vi "createResultsRowLinear.vi"(6 "Indices to Output":bool[](array[boolean]), 7 "Analysis Info cluster":T2[](array[typedef]) {"Sync Delay Time (s)" format="%.4f"; "Total Meas Time (s)" format="%_5g"; "Sd Error in Variance" format="%_3g"; "Skew_u" format="%_3g"; "% u'/U" format="%_3g"; "Sd Error in Mean" format="%_3g"; "Kurt_u" format="%_3g"; "u^4" format="%_3g"; "u^3" format="%_3g"; "U" format="%_3g"; "u^2" format="%_3g"}, 8 "Error String":string, 9 "MetadataValuesIn":string[](array[string]), 11 "MetadataNamesIn":string[](array[string])) -> (0 "row splitting":string[][](array[string]), 1 "Ch Values Out":string[](array[string]), 3 "Ch Names Out":string[](array[string]), 4 "Values to Keep in Dup rows":bool[](array[boolean]))   [LabVIEW 2022 SP3]
uses:
  Controls/Analysis_info_cluster.ctl
  Controls/Inst_type.ctl
  Controls/Instrument_Array.ctl
  Controls/channelState.ctl
  Globals/Dynamic_call_global.ph.vi
panel:
  out "ScrollableArray":T1(array[cluster])
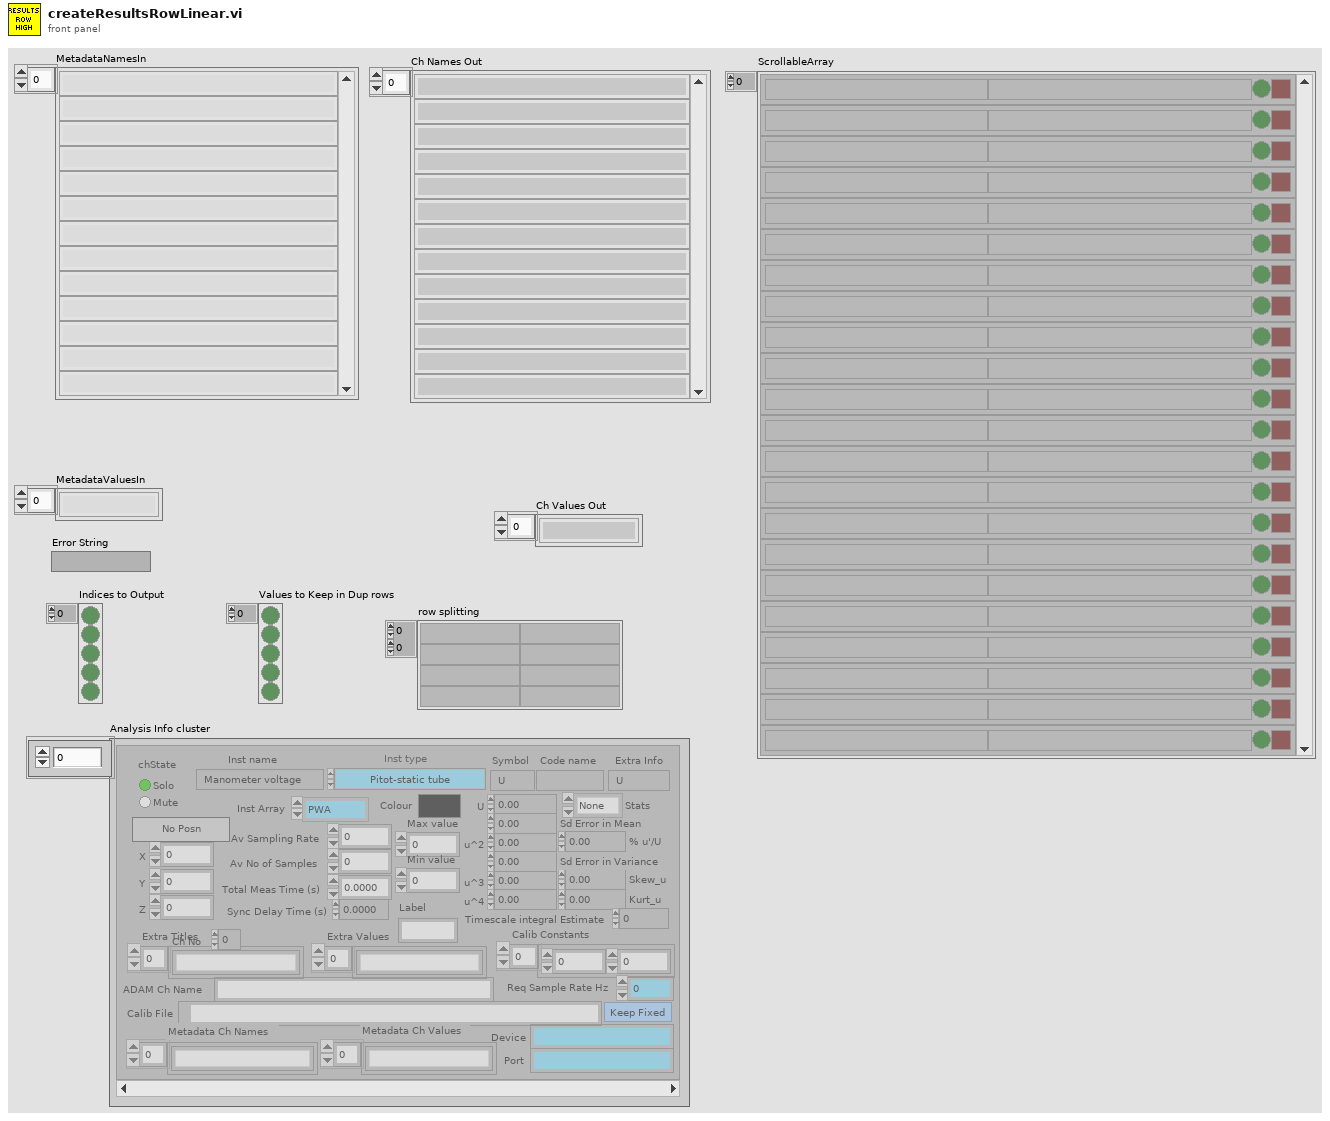
[diagram p1: front panel]
types:
  T1 = cluster{"Input Element":string, "name":string, bool, bool}[]
  T2 = typedef "Analysis_info_cluster.ctl" = cluster{"Colour":u32, "Inst type":T3, "Inst name":string, "Symbol":string, "Code name":string, "Extra Info":string, "Inst Array":T4, "Extra Titles":string[], "Extra Values":string[], "U":dbl, "u^2":dbl, "u^3":dbl, "u^4":dbl, "Skew_u":dbl, "Kurt_u":dbl, "Sd Error in Mean":dbl, "% u'/U":dbl, "X":dbl, "Y":dbl, "Z":dbl, "Timescale integral Estimate":dbl, "Sd Error in Variance":dbl, "Calib File":path, "Calib Constants":dbl[], "Output Position":bool, "Stats":enum16{"None", "Basic", "Full"}, "Av Sampling Rate":dbl, "Av No of Samples":dbl, "Total Meas Time (s)":dbl, "ADAM Ch Name":string, "Max value":dbl, "Min value":dbl, "Req Sample Rate Hz":dbl, "Sync Delay Time (s)":dbl, "Ch No":i16, "Device":string, "Use Latest Calib":bool, "Port":string, "Metadata Ch Names":string[], "Metadata Ch Values":string[], "Label":string, "chState":T5}
  T3 = typedef "Inst_type.ctl" = enum16{"Raw voltage", "Raw with zero offsetting", "Propeller anemometer", "Pressure Transducer", "Pitot-static tube", "Hot wire", "Cross wire 1", "Cross wire 2", "Generic Linear", "Generic Polynomial", "Generic BackPoly", "Fast FID", "Thermocouple", "Cold wire", "Pulsed Wire", "LDA Vel", "LDA Tran time", "LDA Arr time", "Microphone"}
  T4 = typedef "Instrument_Array.ctl" = enum16{"PWA", "LDA", "Analogue"}
  T5 = typedef "channelState.ctl" = enum32{"No Selection", "Solo", "Mute"}
  T6 = cluster{"String":string, "String":string, "Checkbox":bool, bool}
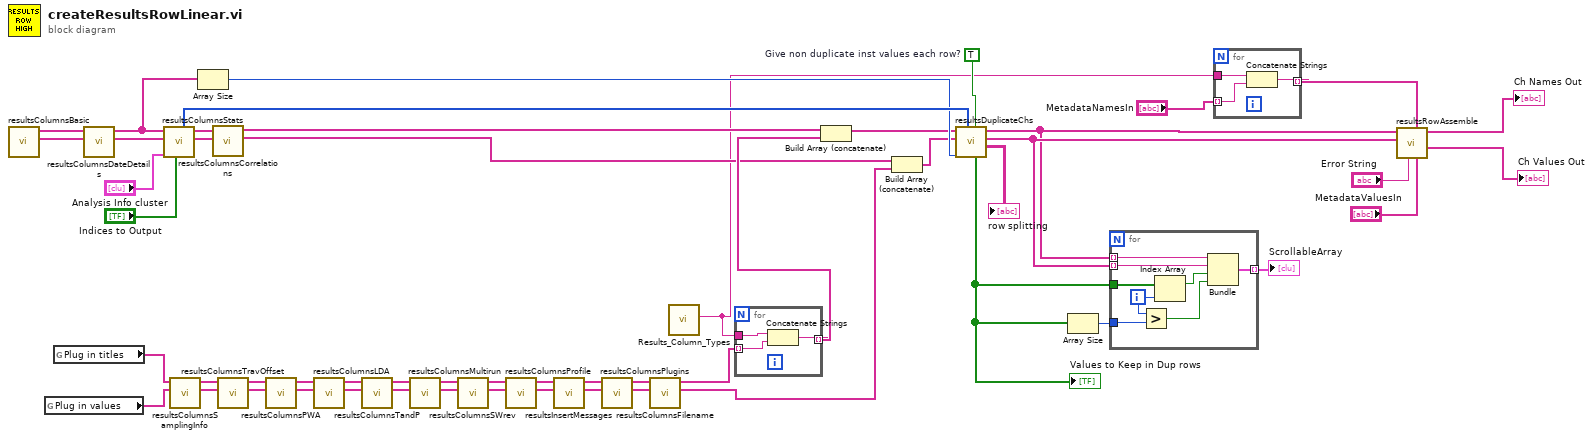
[diagram p0: block diagram]
diagram:
  w36 = TRUE  # Give non duplicate inst values each row?
  n1 = call "resultsColumnsBasic.vi"() -> ("chValues"=w24:string[], "chNames"=w25:string[])  [unwired: 10 in]
  n2 = global read "Dynamic_call_global.ph.vi" "Plug in values"() -> (w13:string[])
  n3 = global read "Dynamic_call_global.ph.vi" "Plug in titles"() -> (w14:string[])
  n4 = call "resultsColumnsDateDetails.vi"("chValuesIn"=w24, "chNamesIn"=w25) -> ("chValuesOut"=w23:string[], "chNamesOut"=w16:string[])  [unwired: 8 in]
  n5 = call "resultsColumnsStats.vi"("Indicies to Output"="Indices to Output", "Analysis Info cluster"="Analysis Info cluster", "chValuesIn"=w23, "chNamesIn"=w16) -> ("chValuesOut"=w46:string[], "chNamesOut"=w47:string[], "dupsArray"=w37:i32[])  [unwired: 5 in]
  n6 = call "resultsColumnsSamplingInfo.vi"("chValuesIn"=w13, "chNamesIn"=w14) -> ("chValuesOut"=w44:string[], "chNamesOut"=w45:string[])  [unwired: 8 in]
  n7 = Array Size(array=w16) -> (size(s)=w15:i32)
  n8 = call "resultsColumnsCorrelations.vi"("chValuesIn"=w46, "chNamesIn"=w47) -> ("chValuesOut"=w4:string[], "chNamesOut"=w8:string[])  [unwired: 8 in]
  n9 = call "resultsColumnsTravOffset.vi"("chValuesIn"=w44, "chNamesIn"=w45) -> ("chValuesOut"=w29:string[], "chNamesOut"=w31:string[])  [unwired: 8 in]
  n10 = call "resultsColumnsPWA.vi"("chValuesIn"=w29, "chNamesIn"=w31) -> ("chValuesOut"=w28:string[], "chNamesOut"=w30:string[])  [unwired: 8 in]
  n11 = call "resultsColumnsLDA.vi"("chValuesIn"=w28, "chNamesIn"=w30) -> ("chValuesOut"=w42:string[], "chNamesOut"=w43:string[])  [unwired: 8 in]
  n12 = call "resultsColumnsTandP.vi"("chValuesIn"=w42, "chNamesIn"=w43) -> ("chValuesOut"=w40:string[], "chNamesOut"=w41:string[])  [unwired: 8 in]
  n13 = call "resultsColumnsMultirun.vi"("chValuesIn"=w40, "chNamesIn"=w41) -> ("chValuesOut"=w21:string[], "chNamesOut"=w22:string[])  [unwired: 8 in]
  n14 = call "resultsColumnsSWrev.vi"("chValuesIn"=w21, "chNamesIn"=w22) -> ("chValuesOut"=w19:string[], "chNamesOut"=w20:string[])  [unwired: 8 in]
  n15 = call "resultsColumnsProfile.vi"("chValuesIn"=w19, "chNamesIn"=w20) -> ("chValuesOut"=w17:string[], "chNamesOut"=w18:string[])  [unwired: 8 in]
  n16 = call "resultsInsertMessages.vi"("chValuesIn"=w17, "chNamesIn"=w18) -> ("chValuesOut"=w26:string[], "chNamesOut"=w27:string[])  [unwired: 8 in]
  n17 = call "resultsColumnsPlugins.vi"("chValuesIn"=w26, "chNamesIn"=w27) -> ("chValuesOut"=w38:string[], "chNamesOut"=w39:string[])  [unwired: 8 in]
  n18 = call "resultsColumnsFilename.vi"("chValuesIn"=w38, "chNamesIn"=w39) -> ("chValuesOut"=w5:string[], "chNamesOut"=w10:string[])  [unwired: 8 in]
  n19 = call "Results_Column_Types.vi"() -> ("Metadata"=w3:string)  [unwired: 9 in, 2 out]
  n20 = for {
    tunnel: w10 -> [w56] mode=indexing
    tunnel: [w55] -> w9 mode=indexing
    tunnel: w3 -> [w54]
    n21 = Concatenate Strings(w54, w56) -> (w55:string)
  }
  n22 = Build Array (concatenate)(w8, w9) -> (w7:string[])
  n23 = Build Array (concatenate)(w4, w5) -> (w6:string[])
  n24 = call "resultsDuplicateChs.vi"("Give non duplicate inst values each row?"=w36, "dupsArray"=w37, "Number of Initial Channels"=w15, "chValuesIn"=w6, "chNamesIn"=w7) -> ("rowSplitting"=→"row splitting":string[][], "chValuesOut"=w12:string[], "chNamesOut"=w11:string[], "valsToKeepinDups"=w33:bool[])  [unwired: 3 in]
  "Values to Keep in Dup rows" <- w33
  n25 = Array Size(array=w33) -> (size(s)=w49:i32)
  n26 = for {
    tunnel: w11 -> [w64] mode=indexing
    tunnel: w12 -> [w63] mode=indexing
    tunnel: w33 -> [w62]
    tunnel: [w61] -> w48 mode=indexing
    tunnel: w49 -> [w58]
    i -> [w59]
    n27 = Greater?(x=w59, y=w58) -> (0:w57:bool)
    n28 = Index Array(array=w62, index=w59) -> (element=w60:bool)
    n29 = Bundle("String"=w64, "String"=w63, "Checkbox"=w60, w57) -> (w61:T6)  [unwired: 1 in]
  }
  "ScrollableArray" <- w48
  n30 = for {
    tunnel: w3 -> [w66]
    tunnel: [w67] -> w1 mode=indexing
    tunnel: "MetadataNamesIn" -> [w65] mode=indexing
    n31 = Concatenate Strings(w66, w65) -> (w67:string)
  }
  n32 = call "resultsRowAssemble.vi"("Ch Values In"="MetadataValuesIn", "Ch Names In"=w1, "ErrorStringIn"="Error String", "RowChValuesIn"=w12, "RowChNamesIn"=w11) -> ("RowChValuesOut"=→"Ch Values Out":string[], "rowChNamesOut"=→"Ch Names Out":string[])  [unwired: 5 in]
